vi "macro_CallbackHelp_MatrixMult_CoerceSizeB.vi"   [LabVIEW 2019, in "Trajectory_Library.lvlib"]
uses:
  MatBuilder_Create.vi
  Trajectory_Library.lvlib
  CallbackHelp_MatrixMult_CoerceSizeB.vi
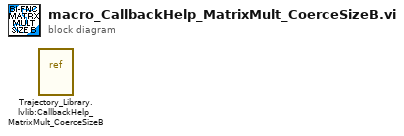
[diagram p0: block diagram]
diagram:
  n1 = vi-ref "Trajectory_Library.lvlib:CallbackHelp_MatrixMult_CoerceSizeB.vi"() -> ()  [unwired: 1 out]
